vi "Timeout.vi"(8 "error in (no error)":errorcluster, 11 "Transfer Line in":refnum<class "Transfer Line.lvclass">) -> (0 "error out":errorcluster, 3 "Transfer Line out":refnum<class "Transfer Line.lvclass">)   [LabVIEW 2015, in "cRIO-Carbondioxide.lvlib" / "CO2-Actor.lvlib" / "Transfer Line.lvclass"]
uses:
  Transfer Line.lvclass
  CO2 Actor/CO2 Actor.lvclass
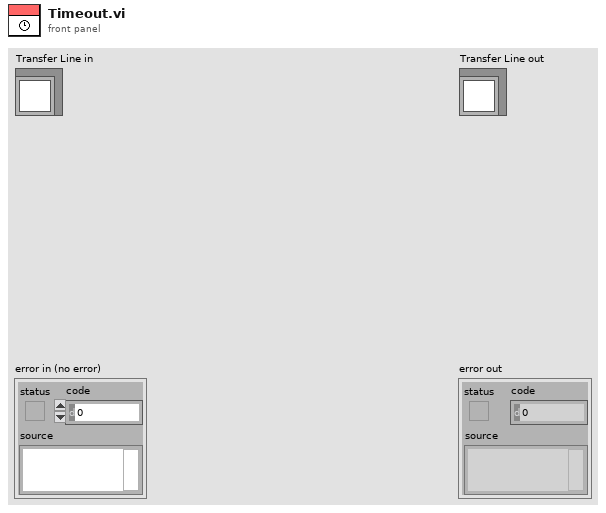
[diagram p1: front panel]
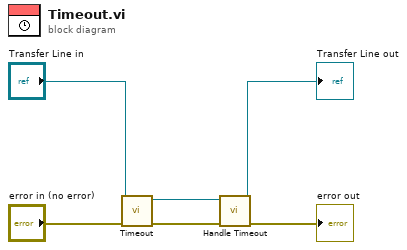
[diagram p0: block diagram]
diagram:
  n1 = call-parent "Timeout.vi"("error in (no error)"="error in (no error)", "CO2 Actor in"="Transfer Line in") -> ("error out"=w4:errorcluster, "CO2 Actor out"=w3:refnum<class "Transfer Line.lvclass">)  [unwired: 8 in]
  n2 = call "Handle Timeout.vi"("error in (no error)"=w4, "Transfer Line in"=w3) -> ("error out"=→"error out":errorcluster, "Transfer Line out"=→"Transfer Line out":refnum<class "Transfer Line.lvclass">)  [unwired: 8 in]
